vi "ParseScriptForFile.vi"(0 "Tree Ref in":refnum<vi>, 5 "Script Array":string[](array[string]), 11 "error in":errorcluster) -> (4 "Tree Ref out":refnum<vi>, 6 "Script Steps":T1[](array[typedef]), 15 "error out":errorcluster)   [LabVIEW 2010]
doc: "This VI gets the info for each step in the script before it gets written to a file"
uses:
  ScriptStepTypeDef.ctl
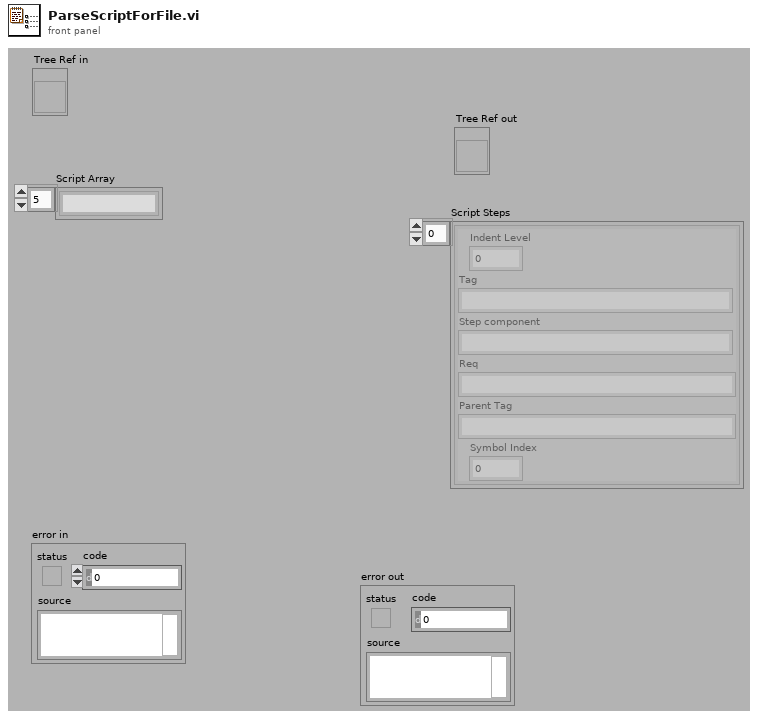
[diagram p1: front panel]
types:
  T1 = typedef "ScriptStepTypeDef.ctl" = cluster{"Indent Level":i32, "Tag":string, "Step component":string, "Req":string, "Parent Tag":string, "Symbol Index":i32}
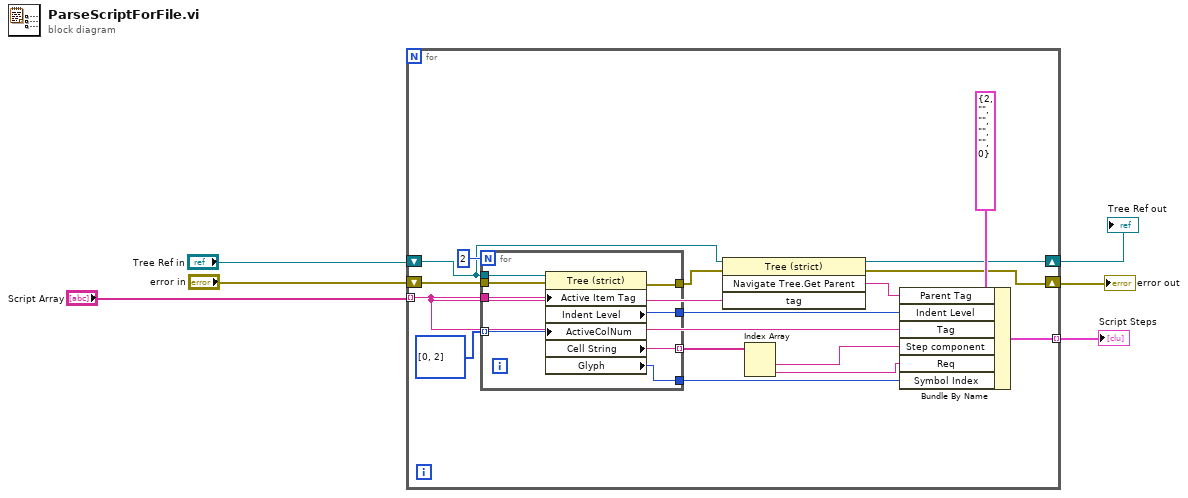
[diagram p0: block diagram]
diagram:
  n1 = for {
    tunnel: "Script Array" -> [w13] mode=indexing
    tunnel: [w21] -> w2 mode=indexing
    shift-right: [w8] -> w1
    shift-left: "Tree Ref in" -> [w14]
    shift-right: [w9] -> w4
    shift-left: "error in" -> [w16]
    n2 = for {
      N: 2 -> [_]
      tunnel: w14 -> [w30]
      tunnel: [w29] -> w12
      tunnel: w13 -> [w28]
      tunnel: [w27] -> w20 mode=indexing
      tunnel: w16 -> [w26]
      tunnel: [w25] -> w10
      tunnel: [w24] -> w15
      tunnel: i32[] [0, 2] -> [w23] mode=indexing
      n3 = property class="Tree (strict)"(reference=w30, error in=w26, "Active Item Tag"=w28, "ActiveColNum"=w23) -> (error out=w25:errorcluster, "Indent Level"=w29:i32, "Cell String"=w27:string, "Glyph"=w24:i32)  [unwired: 1 out]
    }
    n4 = invoke class="Tree (strict)" method="Navigate Tree.Get Parent"(reference=w14, error in=w10, "tag"=w13) -> (reference out=w8:refnum<vi>, error out=w9:errorcluster, "Navigate Tree:Get Parent"=w11:string)  [unwired: 1 in, 1 out]
    n5 = Index Array(array=w20) -> (element #1=w19:string, element #2=w18:string)  [unwired: 2 in]
    n6 = Bundle By Name(cluster=T1 {"Indent Level"=2, "Tag"="", "Step component"="", "Req"="", "Parent Tag"="", "Symbol Index"=0} ("Step"), "Parent Tag"=w11, "Indent Level"=w12, "Tag"=w13, "Step component"=w19, "Req"=w18, "Symbol Index"=w15) -> (w21:T1)
  }
  "error out" <- w4
  "Tree Ref out" <- w1
  "Script Steps" <- w2
